vi "Get Acquisition Timings.vi"(8 "error in (no error)":errorcluster, 9 "kinetic":sgl, 10 "accumulate":sgl, 11 "exposure":sgl) -> (0 "error out":errorcluster, 1 "kinetic out":sgl, 2 "accumulate out":sgl, 3 "exposure out":sgl, 5 "function return":u32)   [LabVIEW 2014, in "atmcd32d.lvlib"]
doc: "unsigned int WINAPI GetAcquisitionTimings(float * exposure, float * accumulate, float * kinetic);"
uses:
  atmcd32d.lvlib
  atmcd32d.dll
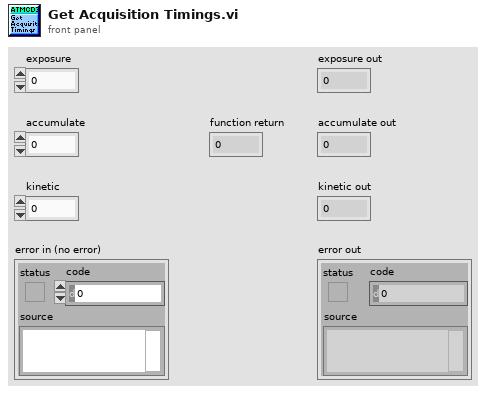
[diagram p1: front panel]
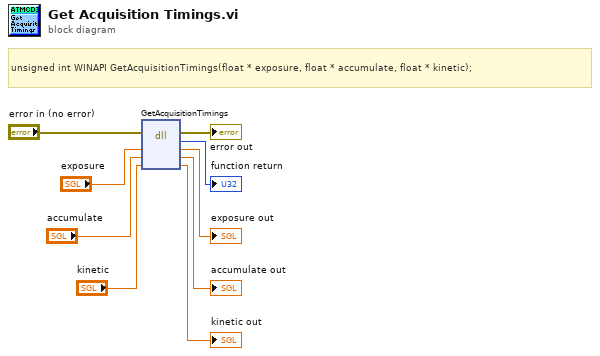
[diagram p0: block diagram]
diagram:
  # "unsigned int WINAPI GetAcquisitionTimings(float * exposure, float * accumulate, float * kinetic);"
  n1 = dll-call lib="C:/Users/Bakir/Documents/Lambda2-Testing/lib/Andorlib/atmcd32d.*" fn="GetAcquisitionTimings"(error in="error in (no error)", "exposure"="exposure", "accumulate"="accumulate", "kinetic"="kinetic") -> (error out=→"error out":errorcluster, →"function return":u32, "exposure"=→"exposure out":sgl, "accumulate"=→"accumulate out":sgl, "kinetic"=→"kinetic out":sgl)  [unwired: 2 in, 1 out]
